vi "6-10.vi"() -> ()   [LabVIEW 2017]
panel:
  out "Waveform Chart":dbl(graph)
  in  "file path (use dialog)":path
  in  "stop":bool
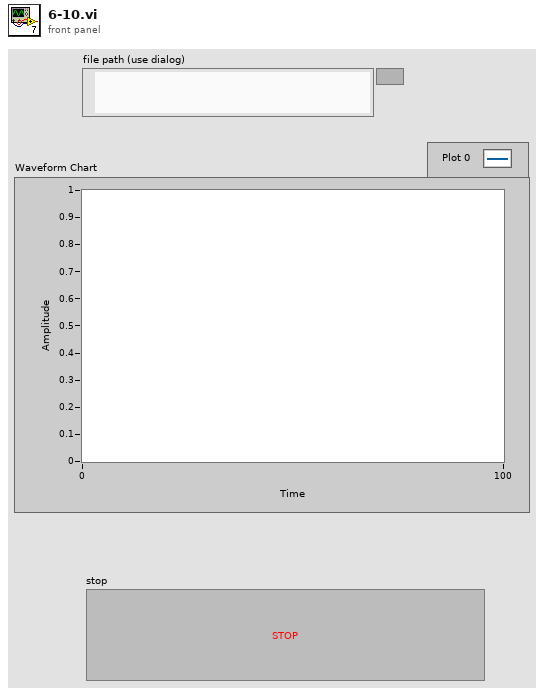
[diagram p1: front panel]
types:
  T1 = enum16{"open", "replace", "create", "open or create", "replace or create", "replace or create with confirmation"}
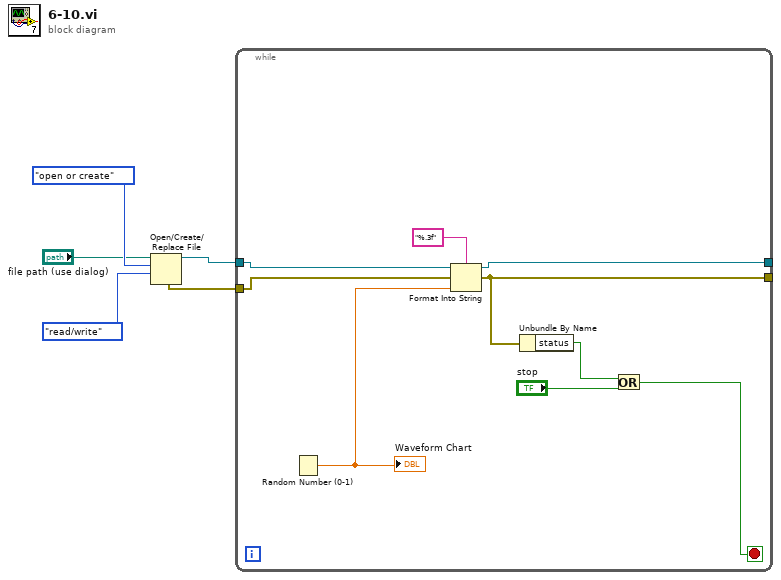
[diagram p0: block diagram]
diagram:
  n1 = Open/Create/Replace File(file path (use dialog)="file path (use dialog)", operation (0:open)=T1."open or create", access (0:read/write)=enum16{"read/write", "read-only", "write-only"}."read/write") -> (refnum out=w5:refnum<file>, error out=w4:errorcluster)  [unwired: 3 in, 1 out]
  n2 = while {
    tunnel: w5 -> [w14]
    tunnel: w4 -> [w13]
    tunnel: [w9] -> _
    tunnel: [w11] -> _
    stop <- w6 stop-if-true
    n3 = Random Number (0-1)() -> (number: 0 to 1=w12:dbl)
    "Waveform Chart" <- w12
    n4 = Format Into String(format string="%.3f", initial string=w14, error in=w13, w12) -> (resulting string=w11:refnum<file>, error out=w9:errorcluster)
    n5 = Unbundle By Name(w9) -> ("status"=w8:bool)
    n6 = Or(x=w8, y="stop") -> (x .or. y?=w6:bool)
  }
